vi "Enum.ConvertToDescription.vi"(8 "error in (no error)":errorcluster, 11 "Enum":variant) -> (0 "error out":errorcluster, 1 "Number":i32[](array[numeric]), 2 "Values":string[](array[string]), 3 "Description":string)   [LabVIEW 2019, in "FPGA Addon System Explorer.lvlib"]
uses:
  FPGA Addon System Explorer.lvlib
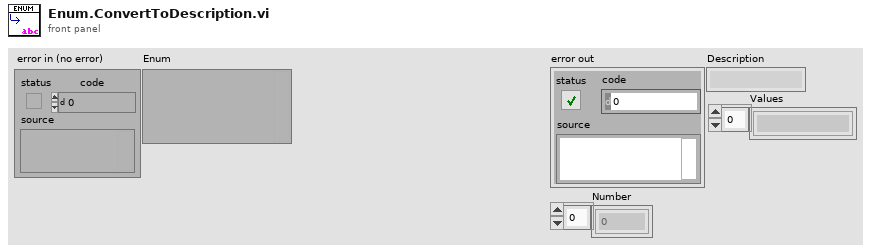
[diagram p1: front panel]
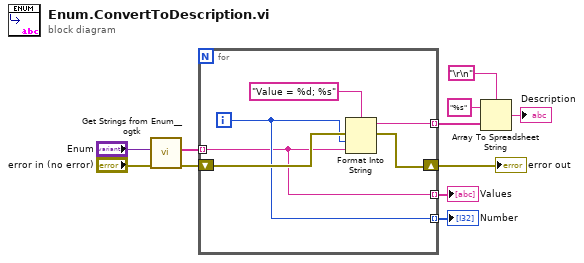
[diagram p0: block diagram]
diagram:
  n1 = call <userlib>:"Get Strings from Enum__ogtk.vi"("error in (no error)"="error in (no error)", "Enum"="Enum") -> ("error out"=w10:errorcluster, "Enum Strings"=w11:string[])  [unwired: 6 in, 2 out]
  n2 = for {
    tunnel: w11 -> [w12] mode=indexing
    tunnel: [w16] -> w6 mode=indexing
    shift-right: [w14] -> w8
    shift-left: w10 -> [w15]
    tunnel: [w13] -> w2 mode=indexing
    tunnel: [w12] -> w1 mode=indexing
    i -> [w13]
    n3 = Format Into String(format string="Value = %d; %s", error in=w15, w13, w12) -> (resulting string=w16:string, error out=w14:errorcluster)  [unwired: 1 in]
  }
  "error out" <- w8
  "Number" <- w2
  "Values" <- w1
  n4 = Array To Spreadsheet String(delimiter (Tab)="\r\n", array=w6, 3:"%s" ("format string")) -> (spreadsheet string=→"Description":string)
